vi "GV input buffer ready.vi"() -> ()   [LabVIEW 2017]
panel:
  in  "Input buffer ready":bool
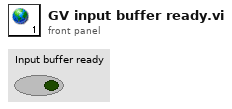
[diagram p1: front panel]
diagram:
